vi "niDAQmx Attach gRPC Task.vi"(8 "error in":errorcluster, 10 "gRPC options":T1={"task name"="", "address (localhost)"="localhost", "port (31763)"=31763}) -> (0 "error out":errorcluster, 3 "task out":refnum<class "Session Factory.lvclass">)   [LabVIEW 2021, in "Session Management niDAQmx.lvlib" / "Session Factory.lvclass"]
doc: "Attaches to an existing niDAQmx task on the specified NI gRPC Device Server. Returns a session factory object to be used in all subsequent niDAQmx client wrapper VI calls."
uses:
  Session Factory.lvclass
  NI DAQmx Client/RPC Messages/nidaqmx_grpc_CreateTaskRequest.ctl
  NI DAQmx Client/RPC Messages/nidevice_grpc_SessionInitializationBehavior.ctl
  Session Factory.lvclass/Session Factory.ctl
  NI DAQmx Client/NI_DAQmx_client.lvlib
  niDAQmx gRPC Device Server.ctl
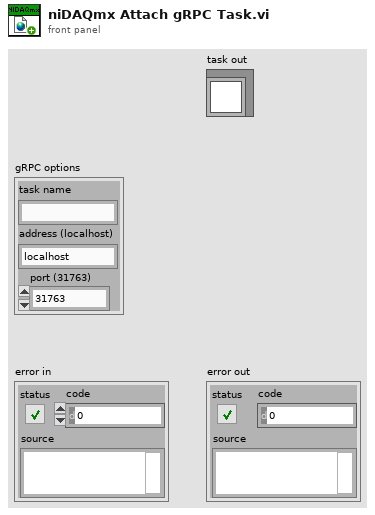
[diagram p1: front panel]
types:
  T1 = typedef "Session Management niDAQmx.lvlib/Session Factory.lvclass/niDAQmx gRPC Device Server.ctl" = cluster{"task name":string, "address (localhost)":string, "port (31763)":u32}
  T2 = typedef "NI_DAQmx_client.lvlib/nidevice_grpc_SessionInitializationBehavior.ctl" = enum32{"SESSION_INITIALIZATION_BEHAVIOR_UNSPECIFIED", "SESSION_INITIALIZATION_BEHAVIOR_INITIALIZE_NEW", "SESSION_INITIALIZATION_BEHAVIOR_ATTACH_TO_EXISTING"}
  T3 = typedef "NI_DAQmx_client.lvlib/nidaqmx_grpc_CreateTaskRequest.ctl" = cluster{"session_name":string, "initialization_behavior":T2}
  T4 = typedef "grpc-lvsupport-release.lvlib/grpcId.ctl" = u64
  T5 = typedef "NI_DAQmx_client.lvlib/nidaqmx_grpc_CreateTaskResponse.ctl" = cluster{"status":i32, "task":T6, "new_session_initialized":bool}
  T6 = typedef "NI_DAQmx_client.lvlib/nidevice_grpc_Session.ctl" = cluster{"nidevice_grpc_Session_session":refnum<class "nidevice_grpc_Session_session.lvclass">}
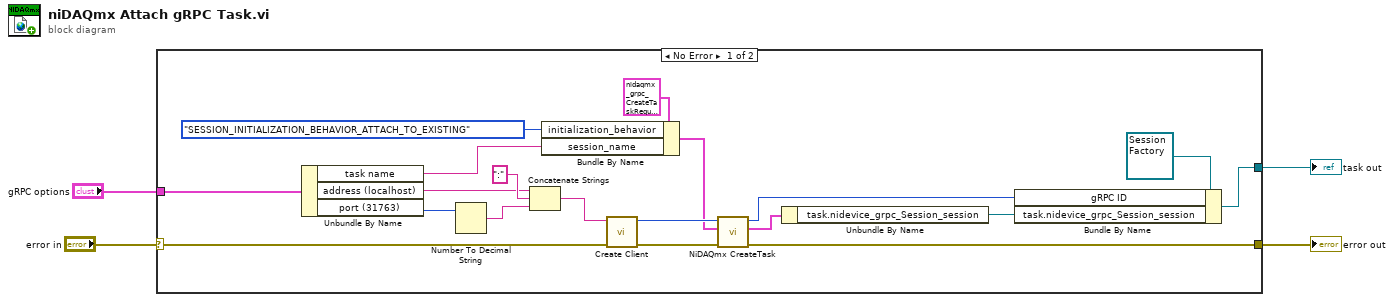
[diagram p0: block diagram]
diagram:
  n1 = case shown="No Error" "error in" {
    selector: "error in" -> [w16 w24]
    tunnel: [w21 w24] -> w3
    tunnel: [w12 _] -> w2
    tunnel: "gRPC options" -> [w10 _]
    frame No Error {
      n2 = Unbundle By Name(w10) -> ("task name"=w9:string, "address (localhost)"=w8:string, "port (31763)"=w7:u32)
      n3 = Number To Decimal String(number=w7) -> (decimal integer string=w6:string)  [unwired: 1 in]
      n4 = Concatenate Strings(w8, ":" ("string"), w6) -> (w19:string)
      n5 = Bundle By Name(cluster=T3 {"session_name"="", "initialization_behavior"=enum."SESSION_INITIALIZATION_BEHAVIOR_INITIALIZE_NEW"} ("Request Data"), "initialization_behavior"=nidevice_grpc_SessionInitializationBehavior."SESSION_INITIALIZATION_BEHAVIOR_ATTACH_TO_EXISTING", "session_name"=w9) -> (w17:T3)
      n6 = call "Create Client.vi"("error in"=w16, "address"=w19) -> ("error out"=w23:errorcluster, "gRPC ID Out"=w22:T4)  [unwired: 8 in]
      n7 = call "NiDAQmx CreateTask.vi"("error in"=w23, "Request Data"=w17, "gRPC ID"=w22) -> ("error out"=w21:errorcluster, "Response Data"=w14:T5, "gRPC ID out"=w15:T4)  [unwired: 6 in]
      n8 = Unbundle By Name(w14) -> ("task.nidevice_grpc_Session_session"=w13:refnum<class "nidevice_grpc_Session_session.lvclass">)
      n9 = Bundle By Name(cluster=refnum<class "Session Factory.lvclass"> refnum ("session factory out"), "gRPC ID"=w15, "task.nidevice_grpc_Session_session"=w13) -> (w12:refnum<class "Session Factory.lvclass">)
    }
    frame Error {
    }
  }
  "error out" <- w3
  "task out" <- w2
